vi "DAQ.DAQmx Find Existing Task.vi"(8 "error in (no error)":errorcluster, 10 "Channels":tag, 11 "Tasks in":refnum<k21>[](array[refnum])) -> (0 "error out":errorcluster, 1 "Task Index":i32, 2 "Channel out":tag, 3 "Task out":refnum<k21>)   [LabVIEW 2019, in "Instrument.Lockin.lvlib" / "Instrument.DAQ.lvclass"]
uses:
  Instrument.DAQ.lvclass
  <resource>/objmgr/daqmx.rc
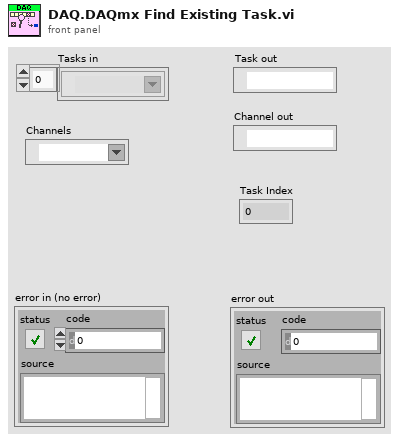
[diagram p1: front panel]
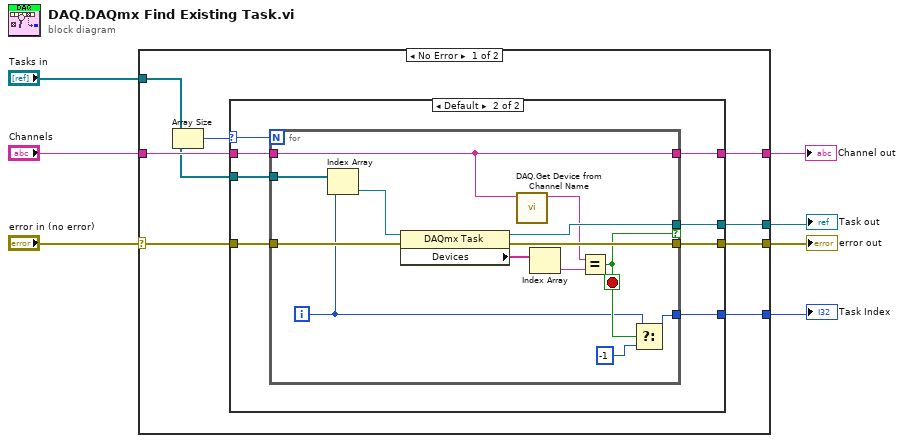
[diagram p0: block diagram]
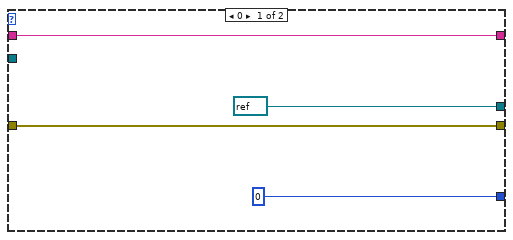
[diagram p2: hidden frame]
diagram:
  n1 = case shown="No Error" "error in (no error)" {
    selector: "error in (no error)" -> [w13 w42]
    tunnel: "Tasks in" -> [w9 _]
    tunnel: "Channels" -> [w14 w41]
    tunnel: [w12 w42] -> w4
    tunnel: [w11 _] -> w3
    tunnel: [w10 _] -> w2
    tunnel: [w8 w41] -> w1
    frame No Error {
      n2 = Array Size(array=w9) -> (size(s)=w15:i32)
      n3 = case shown="Default" w15 {
        selector: w15 -> [_ w25]
        tunnel: w14 -> [w16 w27]
        tunnel: [refnum<k21> refnum ("Refnum out") w26] -> w11
        tunnel: w9 -> [_ w24]
        tunnel: [0 w23] -> w10
        tunnel: w13 -> [w17 w22]
        tunnel: [w17 w21] -> w12
        tunnel: [w16 w20] -> w8
        frame 0 {
        }
        frame Default {
          n4 = for {
            N: w25 -> [_]
            tunnel: w24 -> [w37]
            tunnel: w27 -> [w29]
            tunnel: [w38] -> w26 if=w33
            tunnel: [w30] -> w23
            tunnel: w22 -> [w36]
            tunnel: [w35] -> w21
            tunnel: [w29] -> w20
            i -> [w31]
            stop <- w33 stop-if-true
            n5 = Index Array(array=w37, index=w31) -> (element=w34:refnum<k21>)
            n6 = property class="DAQmx Task"(reference=w34, error in=w36) -> (reference out=w38:refnum<k21>, error out=w35:errorcluster, "Devices"=w40:tag[])
            n7 = call "DAQ.Get Device from Channel Name.vi"("Channel"=w29) -> ("Device"=w28:tag)  [unwired: 10 in]
            n8 = Index Array(array=w40) -> (element=w39:tag)  [unwired: 1 in]
            n9 = Equal?(x=w28, y=w39) -> (x = y?=w33:bool)
            n10 = Select(t=w31, s=w33, f=-1) -> (s? t:f=w30:i32)
          }
        }
      }
    }
    frame Error {
    }
  }
  "error out" <- w4
  "Task Index" <- w2
  "Task out" <- w3
  "Channel out" <- w1
